vi "Image_Crop_Fixed.vi"(8 "Particle Measurements":dbl[][](array[numeric])=[[57.0, 126.0, 60.0, 134.0, 14.0], [248.0, 156.0, 341.0, 306.0, 6231.0], [31.0, 193.0, 32.0, 194.0, 1.0], [324.0, 201.0, 327.0, 209.0, 15.0], [350.0, 252.0, 359.0, 273.0, 108.0], [55.0, 573.0, 56.0, 576.0, 3.0]], 9 "Image  in":T1, 11 "Data":T2={"system"={"info"={"menuSelect"=0, "version"=0, "serial"="Test Sample", "captureActive"=FALSE, "captureBegin"=FALSE, "emptyAndRefill"=FALSE}, "userInfo"={"operatorName"="", "date"=timestamp(2713993200 s since 1904-01-01)}, "camera"={"exposureTime"=0, "aperture"=enum."Item 0", "framerate"=0, "framerateMax"=500, "legacyAttributes"=FALSE}}, "connections"={"arduino"={"connection"="MRJ", "status"=FALSE, "openState"=FALSE, "emptyStart"=0}, "pump"={"connection"="MRJ", "status"=FALSE, "command"="", "dispenseSpeed"=100, "flushSize"=100}, "camera"={"cam1"={"connection"="", "status"=FALSE}, "cam2"={"connection"="", "status"=FALSE}}}, "queue"={"process"={"cam1"=refnum, "cam2"=refnum, "queueSize"=0}, "save"={"cam1"=refnum, "cam2"=refnum, "queueSize"=0}, "overloadThreshold"=0}, "imageProcess"={"cam1"={"preAllocation"={"image"="Station", "originalDisplay"="Station", "originalRgb"="Station", "binary"="Station", "save"="Station", "calibrationFull"=refnum, "calibrationDetect"=refnum}, "calibration"={"pathFull"=path "C:/Users/au540322/Desktop/IHS_Project/images/Debris/Debris_0/Debris_0_2019_06_01-23-32-49-686.PNG", "pathDetect"=path "C:/Users/au540322/Desktop/IHS_Project/images/Debris/Debris_0/Debris_0_2019_06_01-23-32-49-686.PNG", "ROI"={"Left"=0, "Top"=0, "Right"=0, "Bottom"=0, "Rotation"=0.0}}}, "cam2"={"preAllocation"={"image"=refnum, "originalDisplay"=refnum, "originalRgb"=refnum, "binary"=refnum, "save"=refnum, "calibrationFull"=refnum, "calibrationDetect"=refnum}, "calibration"={"pathFull"=path "C:/Users/au540322/Desktop/IHS_Project/images/Debris/Debris_0/Debris_0_2019_06_01-23-32-49-686.PNG", "pathDetect"=path "C:/Users/au540322/Desktop/IHS_Project/images/Debris/Debris_0/Debris_0_2019_06_01-23-32-49-686.PNG", "ROI"={"Left"=0, "Top"=0, "Right"=0, "Bottom"=0, "Rotation"=0.0}}}, "process"={"planeExtract"=refnum, "planeSubtract"=refnum, "cropMask"=refnum}, "detection"={"sampleTimeout"=500, "sizeThreshold"=500, "detectionRegionPct"=0.0}}, "sampleData"={"sampleId"="", "projectId"="", "voucherID"="", "speciesName"="", "collectionDate"=timestamp(2713993200 s since 1904-01-01), "sampleStation"="", "location"="", "lat"=0.0, "lon"=0.0, "determiner"="", "sex"="", "otherNotes"=""}, "Session In"=""} {"sampleData"."collectionDate" format="%<%Y-%m-%d>T"; "imageProcess"."detection"."sizeThreshold" min=1; "imageProcess"."cam2"."calibration"."ROI"."Rotation" format="%.2f"; "imageProcess"."cam2"."calibration"."ROI"."Left" scale=0.0..1024.0; "imageProcess"."cam2"."calibration"."ROI"."Right" scale=0.0..1024.0; "imageProcess"."cam1"."calibration"."ROI"."Rotation" format="%.2f"; "imageProcess"."cam1"."calibration"."ROI"."Left" scale=0.0..1024.0; "imageProcess"."cam1"."calibration"."ROI"."Right" scale=0.0..1024.0; "queue"."overloadThreshold" min=1; "queue"."save"."queueSize" min=1; "queue"."process"."queueSize" min=1; "connections"."pump"."flushSize" min=1; "connections"."pump"."dispenseSpeed" min=1; "system"."camera"."framerateMax" min=1; "system"."userInfo"."date" format="%<%Y-%m-%dT%H:%M:%S+%z>T"; "system"."info"."version" items=["Standard", "XL"]; "system"."info"."menuSelect" items=["Session Data", "Extended Setup", "Buffer", "Camera", "Dispenser", "Stats", "Connections"]}) -> (0 "ROI descriptor":T5={"Global Rectangle"=[233, 141, 356, 321], "Contours"=[{"ID"=enum."External", "Type"=3, "Coordinates"=[233, 141, 356, 321]}]}, 2 "Object accept":bool=TRUE, 3 "Object":bool)   [LabVIEW 2022 SP3]
uses:
  controls/Data.ctl
  <vilib>/userdefined/High Color/IMAQdx.ctl
  <vilib>/vision/Image Controls.llb/IMAQ Image.ctl
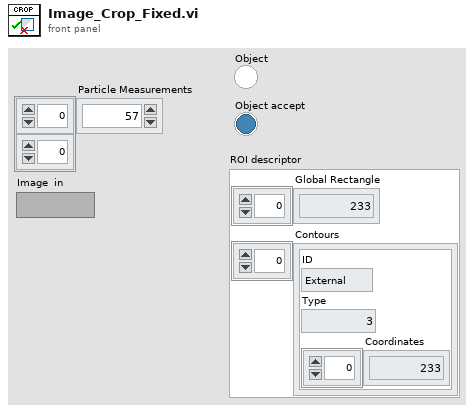
[diagram p1: front panel]
types:
  T1 = typedef "IMAQ Image.ctl" = refnum<image>
  T2 = typedef "Data.ctl" = cluster{"system":cluster{"info":cluster{"menuSelect":u16, "version":u16, "serial":string, "captureActive":bool, "captureBegin":bool, "emptyAndRefill":bool}, "userInfo":cluster{"operatorName":string, "date":timestamp}, "camera":cluster{"exposureTime":i32, "aperture":enum32{"Item 0", "Item 1", "Item 2", "Item 3"}, "framerate":i32, "framerateMax":i32, "legacyAttributes":bool}}, "connections":cluster{"arduino":cluster{"connection":refnum<visa-resource-name>, "status":bool, "openState":bool, "emptyStart":u32}, "pump":cluster{"connection":refnum<visa-resource-name>, "status":bool, "command":string, "dispenseSpeed":i32, "flushSize":i32}, "camera":cluster{"cam1":cluster{"connection":T3, "status":bool}, "cam2":cluster{"connection":T3, "status":bool}}}, "queue":cluster{"process":cluster{"cam1":refnum<queue>, "cam2":refnum<queue>, "queueSize":i32}, "save":cluster{"cam1":refnum<queue>, "cam2":refnum<queue>, "queueSize":i32}, "overloadThreshold":i32}, "imageProcess":cluster{"cam1":cluster{"preAllocation":cluster{"image":T1, "originalDisplay":T1, "originalRgb":T1, "binary":T1, "save":T1, "calibrationFull":T1, "calibrationDetect":T1}, "calibration":cluster{"pathFull":path, "pathDetect":path, "ROI":T4}}, "cam2":cluster{"preAllocation":cluster{"image":T1, "originalDisplay":T1, "originalRgb":T1, "binary":T1, "save":T1, "calibrationFull":T1, "calibrationDetect":T1}, "calibration":cluster{"pathFull":path, "pathDetect":path, "ROI":T4}}, "process":cluster{"planeExtract":T1, "planeSubtract":T1, "cropMask":T1}, "detection":cluster{"sampleTimeout":i32, "sizeThreshold":i32, "detectionRegionPct":dbl}}, "sampleData":cluster{"sampleId":string, "projectId":string, "voucherID":string, "speciesName":string, "collectionDate":timestamp, "sampleStation":string, "location":string, "lat":dbl, "lon":dbl, "determiner":string, "sex":string, "otherNotes":string}, "Session In":T3}
  T3 = typedef "IMAQdx.ctl" = refnum<k21>
  T4 = typedef "IMAQ Rectangle" = cluster{"Left":i32, "Top":i32, "Right":i32, "Bottom":i32, "Rotation":dbl}
  T5 = cluster{"Global Rectangle":i32[], "Contours":cluster{"ID":enum32{"External", "Internal"}, "Type":u32, "Coordinates":i32[]}[]}
  T6 = cluster{"ID":enum32{"External", "Internal"}, "Type":u32, "Coordinates":i32[]}[]
  T7 = cluster{"ID":enum32{"External", "Internal"}, "Type":u32, "Coordinates":i32[]}
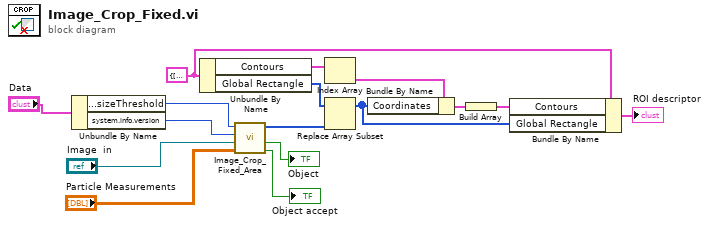
[diagram p0: block diagram]
diagram:
  w9 = T5 {"Global Rectangle"=[106, 29, 356, 265], "Contours"=[{"ID"=enum."External", "Type"=3, "Coordinates"=[106, 29, 356, 265]}]} ("Crop to object")
  n1 = Unbundle By Name("Data") -> ("imageProcess.detection.sizeThreshold"=w7:i32, "system.info.version"=w1:u16)
  n2 = Unbundle By Name(w9) -> ("Contours"=w15:T6, "Global Rectangle"=w16:i32[])
  n3 = call "Image_Crop_Fixed_Area.vi"("Particle Measurements in"="Particle Measurements", "Image  in"="Image  in", "SystemVersion"=w1, "Object size threshold"=w7) -> ("Object accept"=→"Object accept":bool, "Object"=→"Object":bool, "Crop coordinates array"=w8:i32[])  [unwired: 5 in]
  n4 = Index Array(array=w15) -> (element=w14:T7)  [unwired: 1 in]
  n5 = Replace Array Subset(array=w16, new element=w8) -> (w13:i32[])  [unwired: 1 in]
  n6 = Bundle By Name(cluster=w14, "Coordinates"=w13) -> (w12:T7)
  n7 = Build Array(w12) -> (w11:T6)
  n8 = Bundle By Name(cluster=w9, "Contours"=w11, "Global Rectangle"=w13) -> (→"ROI descriptor":T5)
